vi "Get_Map_Cell_Coordinates(SubVI).vi"(8 "error in (no error)":errorcluster, 9 "Y":dbl, 10 "X":dbl) -> (0 "error out":errorcluster, 1 "Y_map":i32, 2 "X_map":i32)   [LabVIEW 2017]
doc: "Convert obstacle double coordinates to map cell position"
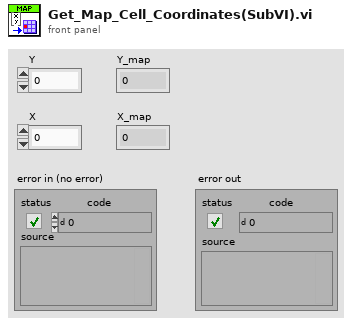
[diagram p1: front panel]
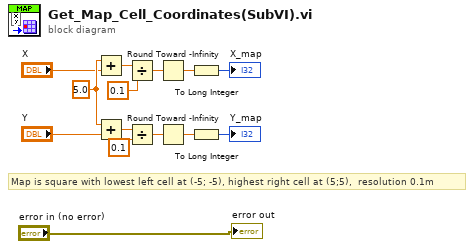
[diagram p0: block diagram]
diagram:
  w12 = 5.0 ("x")
  # "Map is square with lowest left cell at (-5; -5), highest right cell at (5;5),  resolution 0.1m"
  n1 = Add(x=w12, y="X") -> (x+y=w4:dbl)
  n2 = Add(x=w12, y="Y") -> (x+y=w2:dbl)
  n3 = Divide(x=w4, y=0.1) -> (x/y=w13:dbl)
  n4 = Divide(x=w2, y=0.1) -> (x/y=w14:dbl)
  n5 = Round Toward -Infinity(1:w13) -> (0:w7:dbl)
  n6 = Round Toward -Infinity(1:w14) -> (0:w6:dbl)
  n7 = To Long Integer(number=w7) -> (32bit integer=→"X_map":i32)
  n8 = To Long Integer(number=w6) -> (32bit integer=→"Y_map":i32)
  "error out" <- "error in (no error)"
